vi "SET Data.vi"(8 "error in (no error)":errorcluster, 10 "Data":T1={"Text Visible?"=FALSE, "Text Opacity"=0, "Templ Visible?"=FALSE, "Templ Opacity"=0, "Relative Path from 1 to 2"=path "", "Image"=bytes[0], "All User Layers"=[], "Body Text"={"Line 1 text"="", "Line 2 text"="", "Line 3 text"="", "Line 4 text"="", "Line 1 color"=0, "Line 2 color"=0, "Line 3 color"=0, "Line 4 color"=0, "Body Text Spec"={"Font"="", "Alignment"=0, "Size"=3}, "Center text vertically"=FALSE, "Capitalize Text"=FALSE}} {"Body Text"."Body Text Spec"."Alignment" items=["left", "center", "right"]}, 11 "Load & Unload.lvclass in":refnum<class "Load & Unload.lvclass">) -> (0 "error out":errorcluster, 3 "Load & Unload.lvclass out":refnum<class "Load & Unload.lvclass">)   [LabVIEW 2017, in "Load & Unload.lvclass"]
doc: "Sets the class data."
uses:
  <vilib>/LabVIEW Icon API/lv_icon/Classes/Load_Unload/Load & Unload.lvclass
  <vilib>/LabVIEW Icon API/lv_icon/Controls/LabVIEW Icon Stored Information.ctl
  <vilib>/LabVIEW Icon API/lv_icon/Classes/Layer/Layer.lvclass
  <vilib>/LabVIEW Icon API/lv_icon/Controls/BodyText.ctl
  <vilib>/LabVIEW Icon API/lv_icon/Controls/Font.ctl
  <vilib>/LabVIEW Icon API/lv_icon/Controls/Alignment.ctl
  <vilib>/LabVIEW Icon API/lv_icon/Classes/Load_Unload/Load & Unload.lvclass/Load & Unload.ctl
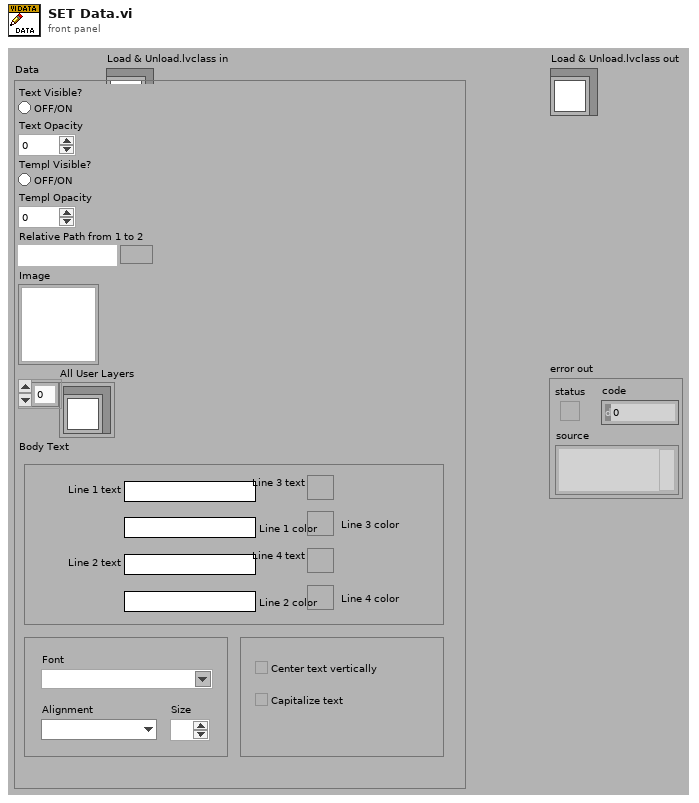
[diagram p1: front panel]
types:
  T1 = typedef "LabVIEW Icon Stored Information.ctl" = cluster{"Text Visible?":bool, "Text Opacity":u8, "Templ Visible?":bool, "Templ Opacity":u8, "Relative Path from 1 to 2":path, "Image":picture, "All User Layers":refnum<class "Layer.lvclass">[], "Body Text":T2}
  T2 = typedef "BodyText.ctl" = cluster{"Line 1 text":string, "Line 2 text":string, "Line 3 text":string, "Line 4 text":string, "Line 1 color":u32, "Line 2 color":u32, "Line 3 color":u32, "Line 4 color":u32, "Body Text Spec":cluster{"Font":T3, "Alignment":T4, "Size":u8}, "Center text vertically":bool, "Capitalize Text":bool}
  T3 = typedef "Font.ctl" = string
  T4 = typedef "Alignment.ctl" = u16
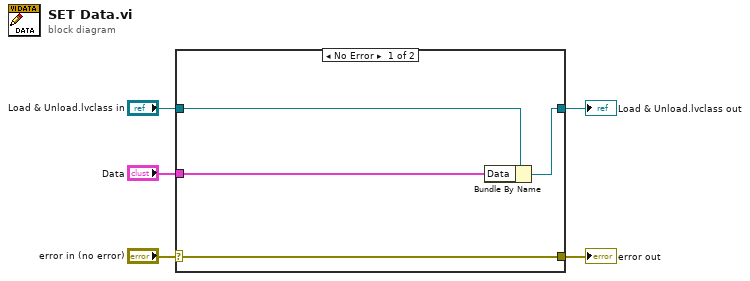
[diagram p0: block diagram]
diagram:
  n1 = case shown="No Error" "error in (no error)" {
    selector: "error in (no error)" -> [w9 w10]
    tunnel: [w9 w10] -> w4
    tunnel: [w7 w11] -> w2
    tunnel: "Load & Unload.lvclass in" -> [w8 w11]
    tunnel: "Data" -> [w6 _]
    frame No Error {
      n2 = Bundle By Name(cluster=w8, "Data"=w6) -> (w7:refnum<class "Load & Unload.lvclass">)
    }
    frame Error {
    }
  }
  "error out" <- w4
  "Load & Unload.lvclass out" <- w2
